vi "Save To Excel.vi"(6 "Excel Template":path, 7 "Output Summary Display":T1 {"Total Energy (W-hr)" format="%#.6g"; "HP Recovery Time (min)" format="%#.4g"; "Mid Run Evap Temp" format="%#.3g"; "Final Discharge Temp" format="%#.3g"; "EEV" format="%#_4g"; "Evap Superheat" format="%#.3g"; "Final Tank Gradient" format="%#.3g"; "UE Max Overshoot" format="%#.3g"; "Temp Drift After Recovery" format="%#.3g"; "Ambient Thermistor Accuracy" format="%#.3g"; "Water Temp Accuracy" format="%#.3g"; "Large Draw Detection" format="%#.3g"; "Gallon @ Compressor ON\nOr Time Value (Minutes)" format="%#.3g"}, 8 "error in (no error)":errorcluster, 9 "HeatUp Data":string[][](array[string])) -> (0 "error out":errorcluster)   [LabVIEW 2016]
uses:
  Type Definitions/Output Summary.ctl
  Type Definitions/HEWH_Type.ctl
  <vilib>/addons/_office/_exclsub.llb/font.ctl
  <vilib>/addons/_office/excel.llb/Excel Easy Table (str).vi
  <vilib>/Utility/NIReport.llb/NI_report.lvclass
  <vilib>/addons/_office/NI_ReportGenerationToolkit.lvlib
  <vilib>/Utility/NIReport.llb/Excel/NI_Excel.lvclass
panel:
  out "error out 2":errorcluster
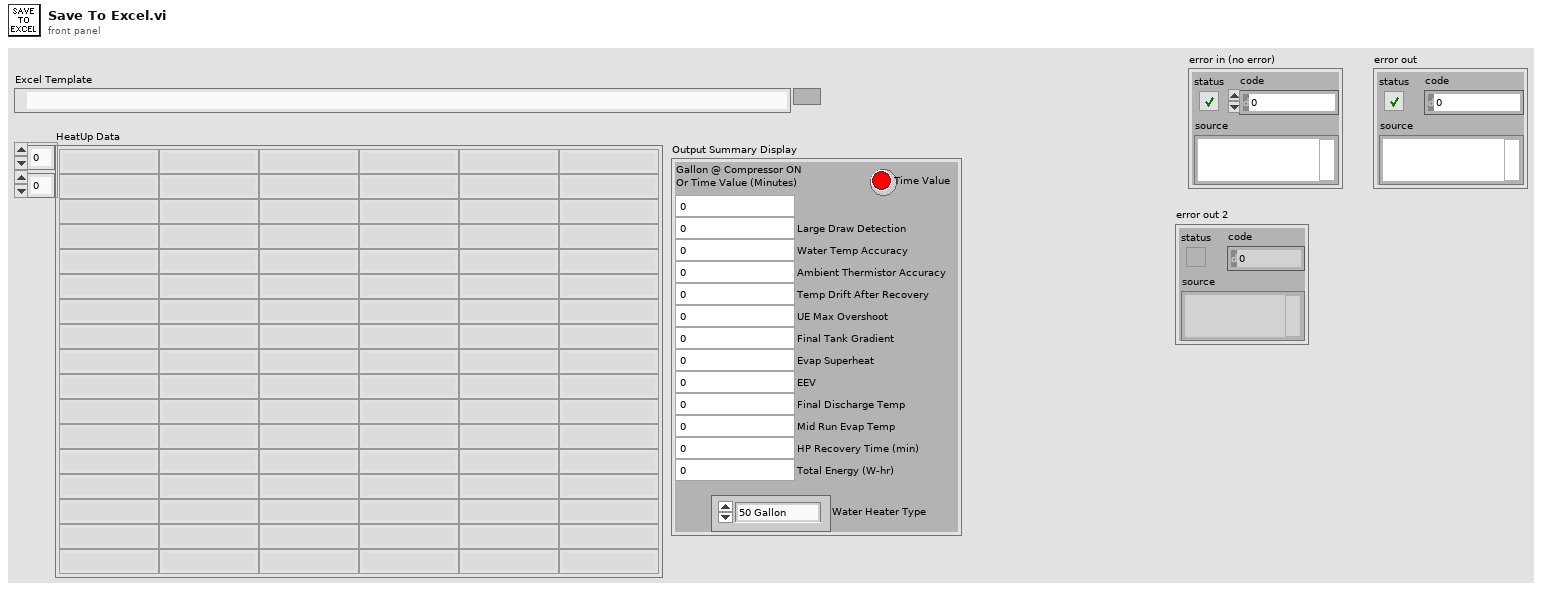
[diagram p1: front panel]
types:
  T1 = typedef "Output Summary.ctl" = cluster{"Gallon @ Compressor ON\nOr Time Value (Minutes)":dbl, "Time Value":bool, "Large Draw Detection":dbl, "Water Temp Accuracy":dbl, "Ambient Thermistor Accuracy":dbl, "Temp Drift After Recovery":dbl, "UE Max Overshoot":dbl, "Final Tank Gradient":dbl, "Evap Superheat":dbl, "EEV":u32, "Final Discharge Temp":dbl, "Mid Run Evap Temp":dbl, "HP Recovery Time (min)":dbl, "Total Energy (W-hr)":dbl, "Water Heater Type":T2}
  T2 = typedef "HEWH_Type.ctl" = enum16{"50 Gallon", "80 Gallon"}
  T3 = cluster{"on/off":bool, "weight":i32, "color":u32}
  T4 = typedef "NI_ReportGenerationToolkit.lvlib/font.ctl" = cluster{"font name":string, "font size":dbl, "bold":u16, "italic":u16, "underline":u16, "strike through":u16, "font color":u32}
  T5 = enum16{"maximized", "minimized", "normal", "no change"}
  T6 = enum16{"Standard Report", "HTML", "Word", "Excel"}
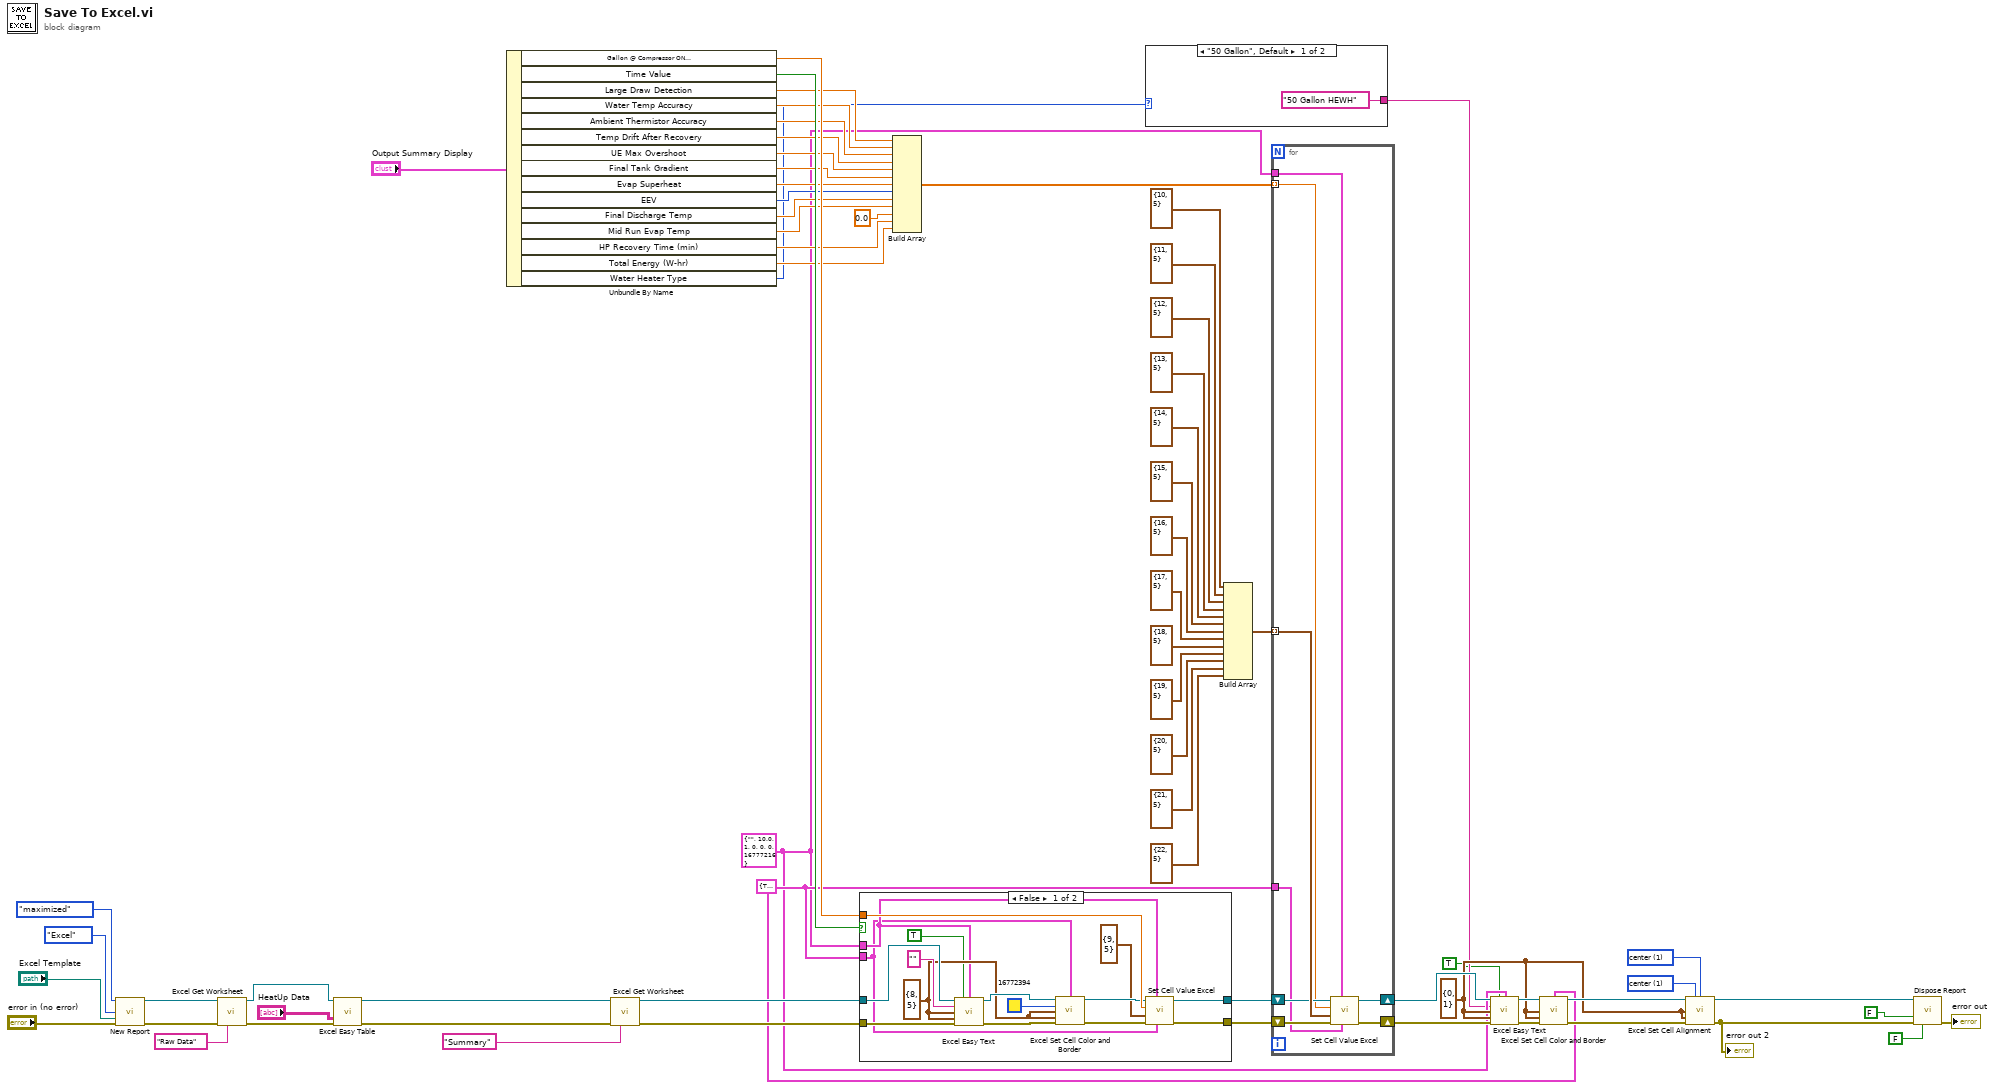
[diagram p0: block diagram]
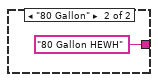
[diagram p2: hidden frame]
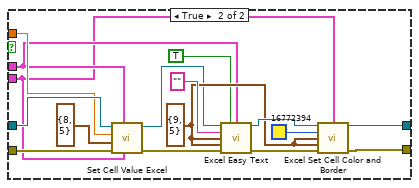
[diagram p3: hidden frame]
diagram:
  w7 = 1 items=["left", "center", "right"] ("horizontal alignment (left)")
  w8 = 1 items=["top", "center", "bottom"] ("vertical alignment (top)")
  w11 = cluster{"row":i32, "column":i32} {"row"=0, "column"=1} ("start (-1, -1)")
  w10 = T3 {"on/off"=TRUE, "weight"=2, "color"=0} ("outside border")
  w9 = T4 {"font name"="", "font size"=10.0, "bold"=1, "italic"=0, "underline"=0, "strike through"=0, "font color"=16777216} ("font")
  n1 = call <vilib>:"New Report.vi"("window state (normal)"=T5."maximized", "report type"=T6."Excel", "template (empty)"="Excel Template", "error in (no error)"="error in (no error)") -> ("report out"=w63:refnum<class "NI_report.lvclass">, "error out"=w64:errorcluster)  [unwired: 10 in]
  n2 = call <vilib>:"Excel Get Worksheet.vi"("report in"=w63, "error in (no error)"=w64, "name (\"\")"="Raw Data" ("name (\"\")")) -> ("report out"=w65:refnum<class "NI_report.lvclass">, "error out"=w66:errorcluster)  [unwired: 11 in]
  n3 = call-poly <vilib>:"Excel Easy Table.vi"("report in"=w65, "text data"="HeatUp Data", "error in (no error)"=w66) -> ("report out"=w54:refnum<class "NI_report.lvclass">, "error out"=w53:errorcluster)  [unwired: 8 in, 3 out]
  n4 = Unbundle By Name("Output Summary Display") -> ("Gallon @ Compressor ON\nOr Time Value (Minutes)"=w47:dbl, "Time Value"=w48:bool, "Large Draw Detection"=w30:dbl, "Water Temp Accuracy"=w29:dbl, "Ambient Thermistor Accuracy"=w28:dbl, "Temp Drift After Recovery"=w27:dbl, "UE Max Overshoot"=w26:dbl, "Final Tank Gradient"=w25:dbl, "Evap Superheat"=w24:dbl, "EEV"=w23:u32, "Final Discharge Temp"=w22:dbl, "Mid Run Evap Temp"=w21:dbl, "HP Recovery Time (min)"=w20:dbl, "Total Energy (W-hr)"=w19:dbl, "Water Heater Type"=w6:T2)
  n5 = call <vilib>:"Excel Get Worksheet.vi"("report in"=w54, "error in (no error)"=w53, "name (\"\")"="Summary" ("name (\"\")")) -> ("report out"=w51:refnum<class "NI_report.lvclass">, "error out"=w50:errorcluster)  [unwired: 11 in]
  n6 = case shown="False" w48 {
    tunnel: w51 -> [w82 w90]
    tunnel: [w72 w94] -> w32
    tunnel: w50 -> [w81 w92]
    tunnel: [w71 w93] -> w31
    tunnel: w47 -> [w83 w87]
    tunnel: w9 -> [w69 w85]
    tunnel: w10 -> [w68 w84]
    frame False {
      w75 = cluster{"row":i32, "column":i32} {"row"=8, "column"=5} ("end (-1, -1)")
      n7 = call <vilib>:"Excel Easy Text.vi"("report in"=w82, "border? (F)"=TRUE, "font"=w69, "text"="", "start (-1, -1)"=w75, "end (-1, -1)"=w75, "error in (no error)"=w81) -> ("report out"=w79:refnum<class "NI_report.lvclass">, "error out"=w78:errorcluster)  [unwired: 4 in, 3 out]
      n8 = call <vilib>:"Excel Set Cell Color and Border.vi"("report in"=w79, "outside border"=w68, "background color (w)"=u32 16772394, "start (-1, -1)"=w75, "end (-1, -1)"=w75, "error in (no error)"=w78) -> ("report out"=w77:refnum<class "NI_report.lvclass">, "error out"=w76:errorcluster)  [unwired: 8 in]
      n9 = call "Set Cell Value Excel.vi"("outside border"=w68, "font"=w69, "error in (no error)"=w76, "end (-1, -1)"=cluster{"row":i32, "column":i32} {"row"=9, "column"=5}, "Gallon @ Compressor ON\nOr Time Value (Minutes)"=w83, "NI_report in"=w77) -> ("error out"=w71:errorcluster, "NI_report out"=w72:refnum<class "NI_report.lvclass">)  [unwired: 4 in]
    }
    frame True {
      w96 = cluster{"row":i32, "column":i32} {"row"=9, "column"=5} ("start (-1, -1)")
      n10 = call "Set Cell Value Excel.vi"("outside border"=w84, "font"=w85, "error in (no error)"=w92, "end (-1, -1)"=cluster{"row":i32, "column":i32} {"row"=8, "column"=5} ("start (-1, -1)"), "Gallon @ Compressor ON\nOr Time Value (Minutes)"=w87, "NI_report in"=w90) -> ("error out"=w91:errorcluster, "NI_report out"=w89:refnum<class "NI_report.lvclass">)  [unwired: 4 in]
      n11 = call <vilib>:"Excel Easy Text.vi"("report in"=w89, "border? (F)"=TRUE, "font"=w85, "text"="", "start (-1, -1)"=w96, "end (-1, -1)"=w96, "error in (no error)"=w91) -> ("report out"=w98:refnum<class "NI_report.lvclass">, "error out"=w97:errorcluster)  [unwired: 4 in, 3 out]
      n12 = call <vilib>:"Excel Set Cell Color and Border.vi"("report in"=w98, "outside border"=w84, "background color (w)"=u32 16772394, "start (-1, -1)"=w96, "end (-1, -1)"=w96, "error in (no error)"=w97) -> ("report out"=w94:refnum<class "NI_report.lvclass">, "error out"=w93:errorcluster)  [unwired: 8 in]
    }
  }
  n13 = Build Array(w30, w29, w28, w27, w26, w25, w24, w23, w22, w21, 0.0, w20, w19) -> (w18:dbl[])
  n14 = case shown="\"50 Gallon\", Default" w6 {
    tunnel: ["50 Gallon HEWH" "80 Gallon HEWH"] -> w5
    frame "50 Gallon", Default {
    }
    frame "80 Gallon" {
    }
  }
  n15 = Build Array(cluster{"row":i32, "column":i32} {"row"=10, "column"=5} ("end (-1, -1)"), cluster{"row":i32, "column":i32} {"row"=11, "column"=5} ("end (-1, -1)"), cluster{"row":i32, "column":i32} {"row"=12, "column"=5} ("end (-1, -1)"), cluster{"row":i32, "column":i32} {"row"=13, "column"=5} ("end (-1, -1)"), cluster{"row":i32, "column":i32} {"row"=14, "column"=5} ("end (-1, -1)"), cluster{"row":i32, "column":i32} {"row"=15, "column"=5} ("end (-1, -1)"), cluster{"row":i32, "column":i32} {"row"=16, "column"=5} ("end (-1, -1)"), cluster{"row":i32, "column":i32} {"row"=17, "column"=5} ("end (-1, -1)"), cluster{"row":i32, "column":i32} {"row"=18, "column"=5} ("end (-1, -1)"), cluster{"row":i32, "column":i32} {"row"=19, "column"=5} ("end (-1, -1)"), cluster{"row":i32, "column":i32} {"row"=20, "column"=5} ("end (-1, -1)"), cluster{"row":i32, "column":i32} {"row"=21, "column"=5} ("end (-1, -1)"), cluster{"row":i32, "column":i32} {"row"=22, "column"=5} ("end (-1, -1)")) -> (w33:cluster{"row":i32, "column":i32}[])
  n16 = for {
    tunnel: w33 -> [w109] mode=indexing
    shift-right: [w107] -> w13
    shift-left: w32 -> [w108]
    shift-right: [w105] -> w12
    shift-left: w31 -> [w106]
    tunnel: w18 -> [w104] mode=indexing
    tunnel: w9 -> [w103]
    tunnel: w10 -> [w102]
    n17 = call "Set Cell Value Excel.vi"("outside border"=w102, "font"=w103, "error in (no error)"=w106, "end (-1, -1)"=w109, "Gallon @ Compressor ON\nOr Time Value (Minutes)"=w104, "NI_report in"=w108) -> ("error out"=w105:errorcluster, "NI_report out"=w107:refnum<class "NI_report.lvclass">)  [unwired: 4 in]
  }
  n18 = call <vilib>:"Excel Easy Text.vi"("report in"=w13, "border? (F)"=TRUE, "font"=w9, "text"=w5, "start (-1, -1)"=w11, "end (-1, -1)"=w11, "error in (no error)"=w12) -> ("report out"=w17:refnum<class "NI_report.lvclass">, "error out"=w16:errorcluster)  [unwired: 4 in, 3 out]
  n19 = call <vilib>:"Excel Set Cell Color and Border.vi"("report in"=w17, "outside border"=w10, "start (-1, -1)"=w11, "end (-1, -1)"=w11, "error in (no error)"=w16) -> ("report out"=w15:refnum<class "NI_report.lvclass">, "error out"=w14:errorcluster)  [unwired: 9 in]
  n20 = call <vilib>:"Excel Set Cell Alignment.vi"("report in"=w15, "vertical alignment (top)"=w8, "horizontal alignment (left)"=w7, "start (-1, -1)"=w11, "end (-1, -1)"=w11, "error in (no error)"=w14) -> ("report out"=w2:refnum<class "NI_report.lvclass">, "error out"=w1:errorcluster)  [unwired: 8 in]
  "error out 2" <- w1
  n21 = call-dynamic "Dispose Report.vi"("report in"=w2, "save changes? (F)"=FALSE, "error in (no error)"=w1, "close report? (T)"=FALSE) -> ("error out"=→"error out":errorcluster)  [unwired: 11 in]
